vi "Model-free setpoint control0216.vi"() -> ()   [LabVIEW 2018]
doc: "Demonstrates the use of the Network Streams functions to send LED status to the myRIO target."
uses:
  <vilib>/ErrorRing/Error Ring.xnode
  <vilib>/vision/NI_Vision_Development_Module.lvlib
panel:
  in  "base_pr":dbl=-37.75
  in  "base_dr":dbl=-62.3
  in  "K2":dbl=0.109
  in  "K1":dbl=0.138
  in  "Operation":T1(ring)=enum."Erode"
  out "real_relative_point_y":dbl
  out "real_relative_point_x":dbl
  out "real_relative_start_point_y":dbl
  out "real_relative_start_point_x":dbl
  out "Bounding Box.Y Top 2":i32
  out "Bounding Box.X Left 2":i32
  out "Ki part":dbl
  out "Kd part":dbl
  out "Kp part":dbl
  out "Ki part":dbl
  out "Kd part":dbl
  out "Kp part":dbl
  in  "Ki":dbl=0.002
  in  "Kd":dbl=1e-05
  in  "Kp":dbl=0.005
  in  "Ki":dbl=0.002
  in  "Kd":dbl=1e-05
  in  "Kp":dbl=0.005
  out "添加的数组":dbl[](array[numeric])
  in  "desired_relative_point_y":dbl=500.0
  in  "desired_relative_point_x":dbl=400.0
  out "predicted_output_pr":dbl=20.0
  out "predicted_output_dr":dbl=8.0
  out "error_relative_point_y":dbl
  out "error_relative_point_x":dbl
  out "real_relative_end_point_y":dbl
  out "real_relative_end_point_x":dbl
  out "magnet_input_pr":dbl
  out "magnet_input_dr":dbl
  in  "打开仅尖端轨迹":bool
  out "仅尖端轨迹":T2(plugin-control)
  out "Bounding Box.Y Top":i32
  out "Bounding Box.X Left":i32
  out "curve_min_y":dbl
  out "curve_min_x":dbl
  out "curve_max_y":dbl
  out "curve_max_x":dbl
  out "relative_end_point_y":dbl
  out "relative_end_point_x":dbl
  out "delta_y":dbl
  out "delta_x":dbl
  out "pr":dbl
  out "tan(v)":dbl
  out "delta_velocity":dbl format="%#_10g"
  out "delta_time":dbl
  out "now time":timestamp[](array[timestamp])
  out "prev time":timestamp[](array[timestamp])
  out "delta_distance":dbl
  out "prev_end_point_y":dbl
  out "prev_end_point_x":dbl
  out "now_end_point_y":dbl
  out "now_end_point_x":dbl
  out "prev_end_point_y":dbl[](array[numeric])
  out "prev_end_point_x":dbl[](array[numeric])
  out "dr":dbl
  in  "Ar":sgl=11.0
  out "all parameters":dbl[][](array[numeric])
  out "direction angle":sgl[](array[numeric])
  out "dr":sgl
  out "strength":dbl[](array[numeric])
  out "场强":dbl
  out "end_point_y":T3
  out "end_point_x":dbl[](array[numeric])
  out "start_point_y":dbl[](array[numeric])
  out "start_point_x":dbl[](array[numeric])
  out "T":i32[](array[numeric])
  out "c":dbl[](array[numeric])
  out "b":dbl[](array[numeric])
  out "a\na":dbl[](array[numeric])
  out "c":dbl
  out "b":dbl
  out "a":dbl
  out "Angles (deg)":sgl[](array[numeric]) format="%.2f"
  in  "wr":sgl
  in  "打开轨迹":bool
  out "中心轨迹和尖端轨迹":T2(plugin-control)
  out "end_y":dbl
  out "end_x":dbl
  out "start_y":dbl
  out "start_x":dbl
  out "Image Pixels (U8)":u8[][](array[numeric])
  in  "Poly":dbl
  out "中心轨迹":T2(plugin-control)
  in  "保存按钮":bool
  out "Object Center":cluster{"X":sgl, "Y":sgl}
  out "黑白图":T2(plugin-control)
  in  "Number of Erosion":i32=5
  in  "Settings":T4={"Objects"=1, "Threshold"=128, "Reject Border"=FALSE, "Fill Holes"=FALSE, "Min Object Size"=TRUE, "Min Size"=5500, "Max Object Size"=FALSE, "Max Size"=100, "Show Search Area"=TRUE, "Show Center"=TRUE, "Show Bounding Box"=TRUE} {"Objects" items=["Bright Objects", "Dark Objects"]; "Threshold" min=1 max=999999999 step=1; "Max Size" min=1 max=999999999 step=1; "Min Size" min=1 max=999999999 step=1}
  out "Objects":T5(array[cluster]) {"Aspect Ratio" format="%.2f"; "Orientation" format="%.2f"; "Area" format="%.2f"; "Object Center"."Y" format="%.2f"; "Object Center"."X" format="%.2f"}
  in  "Search Rect (entire image)":T6={"Left"=160, "Top"=740, "Right"=1900, "Bottom"=1620, "Rotation"=0.0} {"Rotation" format="%.2f"; "Left" scale=0.0..1024.0; "Right" scale=0.0..1024.0}
  in  "Range":cluster{"Lower value":sgl, "Upper value":sgl}={"Lower value"=170.0, "Upper value"=255.0} {"Upper value" format="%.2f"; "Lower value" format="%.2f"}
  out "原图":T2(plugin-control)
  in  "停止":bool
  out "T":i32
  out "T":i32
  in  "磁场变换":bool=TRUE
  in  "Pause":bool
  out "Array":dbl[](array[numeric])
  in  "Parameter Settings":T7(tab)=enum."Rotating Field" caption="Field Types"
  in  "Ag":dbl
  in  "dg":dbl
  in  "pg":dbl
  in  "fg":dbl
  in  "AoOF":dbl
  in  "fo":sgl
  in  "do":sgl
  in  "oo":sgl
  in  "po":sgl
  in  "cc":sgl
  in  "pc":sgl
  in  "wc":sgl
  in  "dc":sgl
  in  "Ac":dbl
  in  "Dis phase step":dbl
  in  "Dis phase frequency (Hz)":dbl
  in  "Dis tumbling frequency (Hz)":dbl
  in  "Dis strength(mT)":dbl
  in  "Swa strength (mT)":dbl
  in  "Swa frequency (Hz)":dbl
  in  "Swa pitch angle (deg)":dbl
  in  "Swa direction angle (deg)":dbl
  in  "Swa ratio":dbl=1.0
  in  "Pitch Angle (rotating around Constant, deg)":dbl
  in  "Ratio (A/C)":sgl
  in  "Direction Angle (deg)":sgl
  in  "Pitch Angle (rotating around Origin, deg)":sgl
  in  "Frequency (Hz)":sgl
  in  "Strength (mT)":dbl
  in  "Ar 2":dbl caption="Ar"
  in  "ratio":sgl
  in  "pr  2":sgl
  in  "dr  2":sgl
  in  "wr  2":sgl
  in  "p_x":sgl
  out "Numeric 5":i32
  in  "Stop":bool
  out "error out":errorcluster
  in  "Target IP Address":string="172.22.11.2"
  # "Overview: Magnetic field calculation, and send parameters to myRIO\nInstructions:\n1. Verify the value of Target IP Address. Set Visa resource name.\n2. Ensure RT Main.vi is already running. \n3. Run this VI. Set parameters of magnetic field."
  # "Strength (mT)"
  # "Frequency (Hz)"
  # "Pitch Angle (deg)"
  # "Direction Angle (deg)"
  # "Strength (mT)"
  # "Pitch Angle (deg)"
  # "Direction Angle (deg)"
  # "Frequency (Hz)"
  # "Strength (mT)"
  # "Oscilation Frequency (Hz)"
  # "Oscilation Angle (deg)"
  # "Pitch Angle (deg)"
  # "Direction Angle (deg)"
  # "Strength (mT)"
  # "Frequency (Hz)"
  # "Pitch Angle (deg)"
  # "Direction Angle (deg)"
  # "Conical Angle (deg)"
  # "Strength (mT)"
  # "Tumbling Frequency (Hz)"
  # "Phase Frequency (Hz)"
  # "Phase Step"
  # "Strength (mT)"
  # "Frequency (Hz)"
  # "Pitch Angle (deg)"
  # "Direction Angle (deg)"
  # "Ratio"
  # "Strength (mT)"
  # "Frequency (Hz)"
  # "Ratio (A/C)"
  # "Direction Angle (deg)"
  # "Pitch Angle (rotating around Origin, deg)"
  # "Pitch Angle (rotating around Constant, deg)"
  # "Strength (mT)"
  # "Frequency (Hz)"
  # "Pitch Angle Y (deg)"
  # "Pitch Angle X (deg)"
  # "Direction Angle (deg)"
  # "ratio (l/s)"
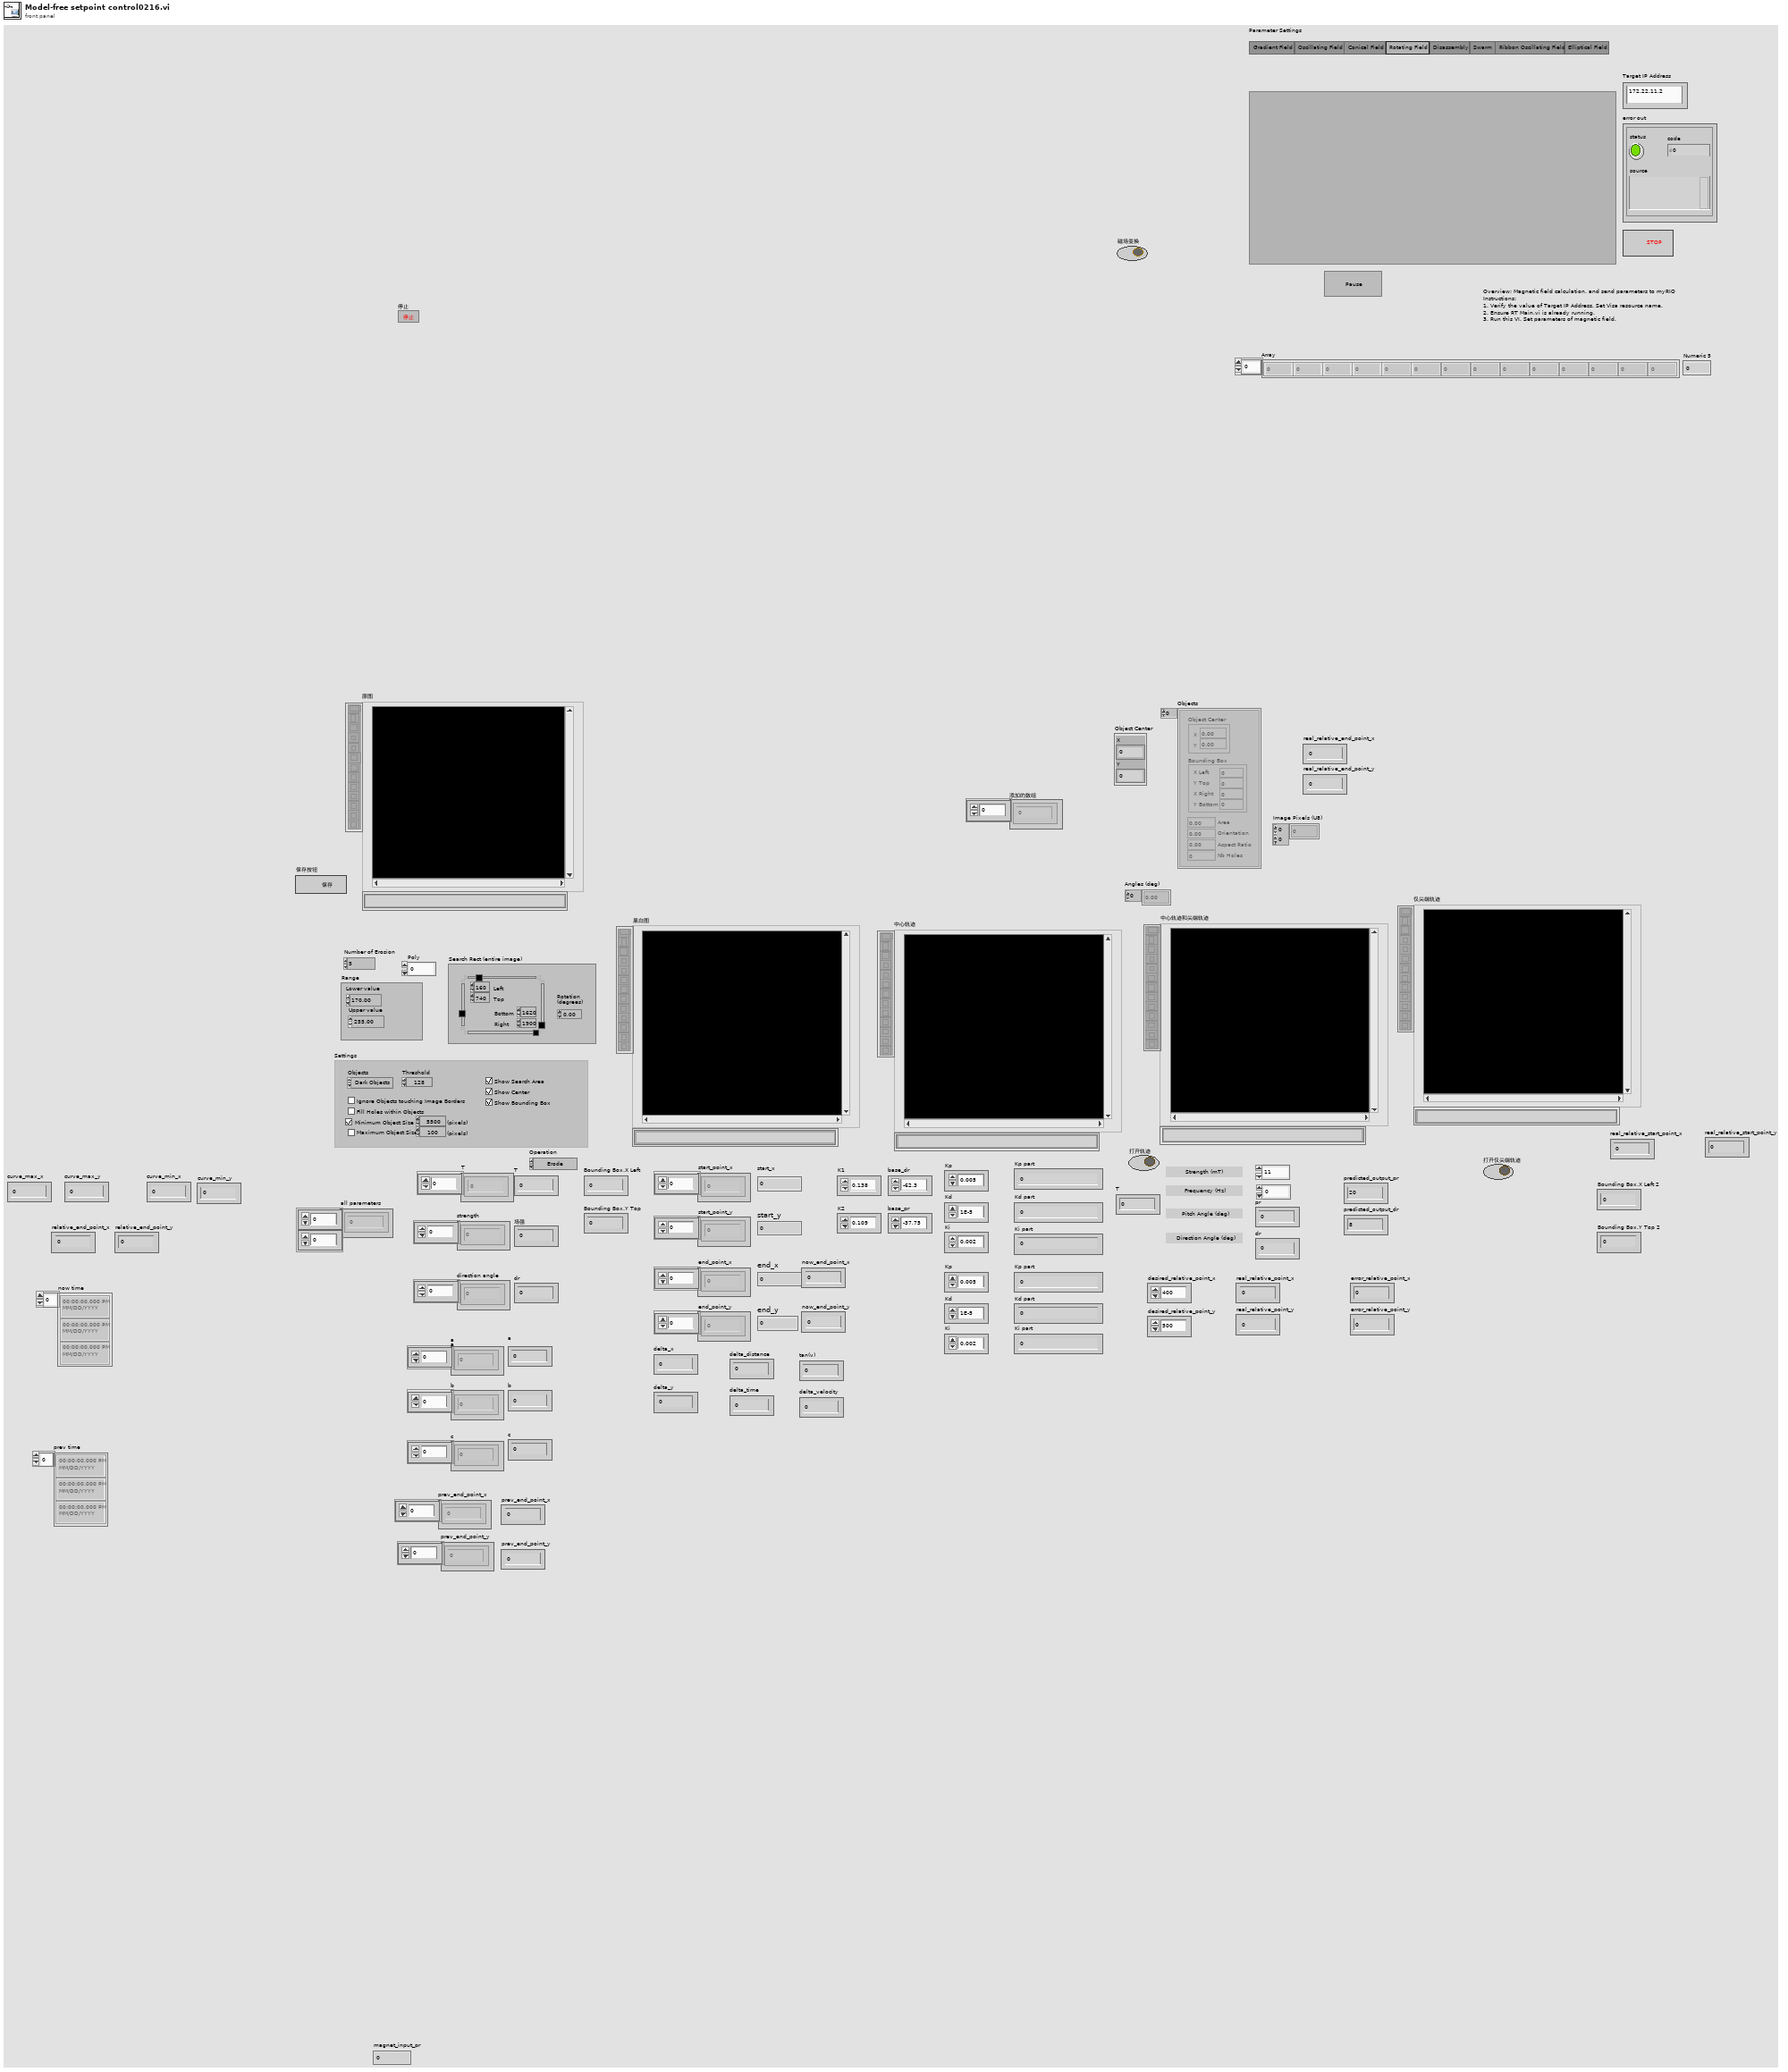
[diagram p1: front panel]
types:
  T1 = enum32{"AutoM", "Close", "Dilate", "Erode", "Gradient", "Gradient in", "Gradient out", "HitMiss", "Open", "PClose", "POpen", "Thick", "Thin"}
  T2 = typedef "IMAQ Image.ctl" = refnum<image>
  T3 = typedef "控件 3.ctl" = dbl[]
  T4 = cluster{"Objects":u16, "Threshold":i32, "Reject Border":bool, "Fill Holes":bool, "Min Object Size":bool, "Min Size":i32, "Max Object Size":bool, "Max Size":i32, "Show Search Area":bool, "Show Center":bool, "Show Bounding Box":bool}
  T5 = cluster{"Object Center":cluster{"X":sgl, "Y":sgl}, "Bounding Box":cluster{"X Left":i32, "Y Top":i32, "X Right":i32, "Y Bottom":i32}, "Area":sgl, "Orientation":sgl, "Aspect Ratio":sgl, "Nb Holes":i32}[]
  T6 = typedef "IMAQ Rectangle" = cluster{"Left":i32, "Top":i32, "Right":i32, "Bottom":i32, "Rotation":dbl}
  T7 = enum32{"Gradient Field ", "Oscillating Field", "Conical Field", "Rotating Field", "Disassembly", "Swarm", "Ribbon Oscillating Field", "Elliptical Field"}
  T8 = typedef "Image Type" = u32
  T9 = cluster{"Object Center":cluster{"X":sgl, "Y":sgl}, "Bounding Box":cluster{"X Left":i32, "Y Top":i32, "X Right":i32, "Y Bottom":i32}, "Area":sgl, "Orientation":sgl, "Aspect Ratio":sgl, "Nb Holes":i32}
  T10 = cluster{"X Left":i32, "Y Top":i32, "X Right":i32, "Y Bottom":i32, "Rotation":dbl}
  T11 = typedef "ROI Descriptor" = cluster{"Global Rectangle":i32[], "Contours":cluster{"ID":enum32{"External", "Internal"}, "Type":u32, "Coordinates":i32[]}[]}
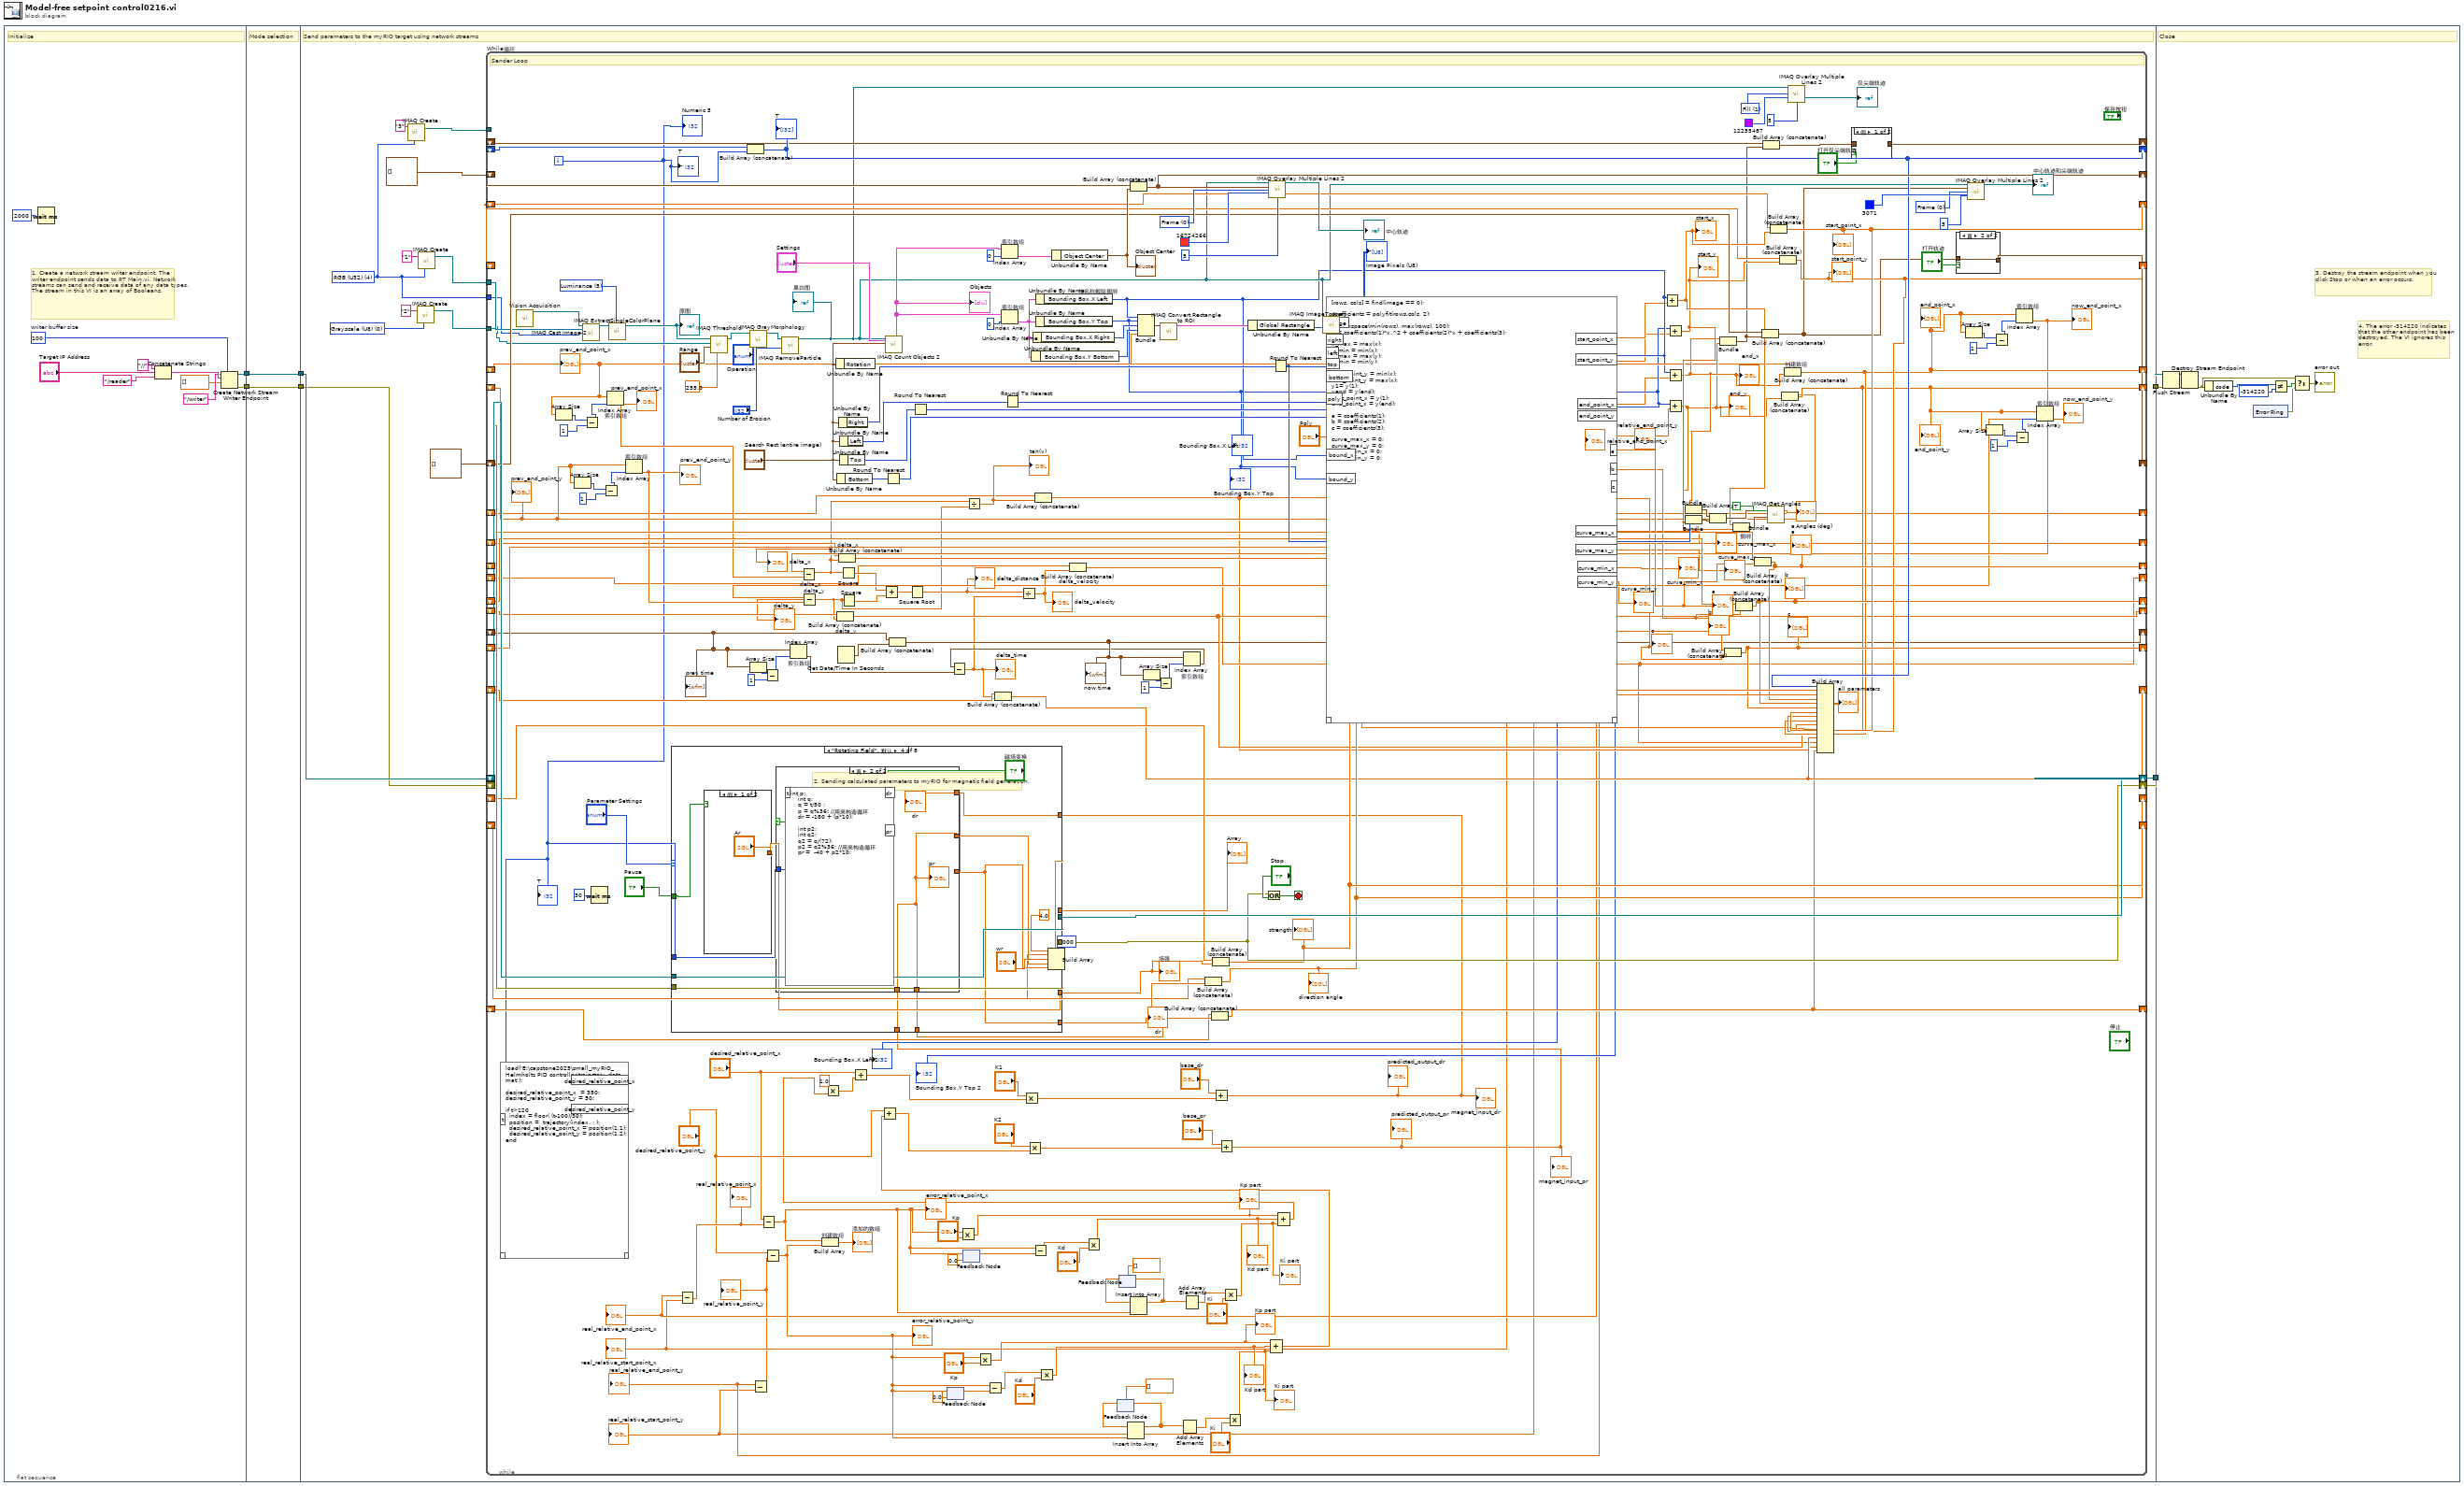
[diagram p0: block diagram]
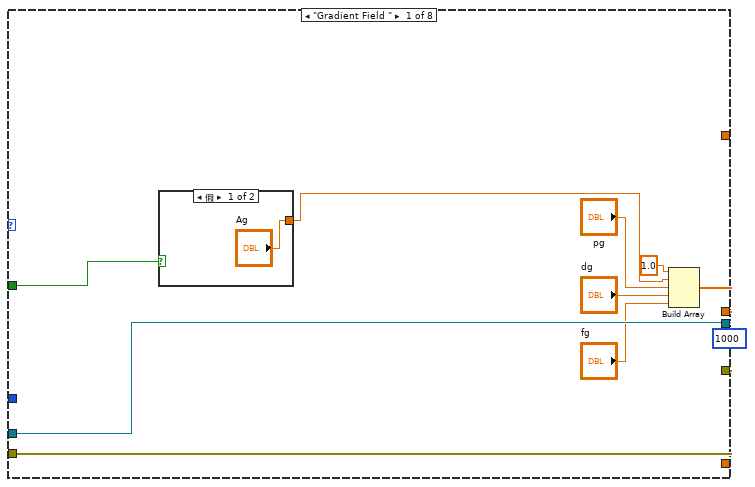
[diagram p4: hidden frame]
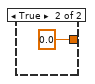
[diagram p5: hidden frame]
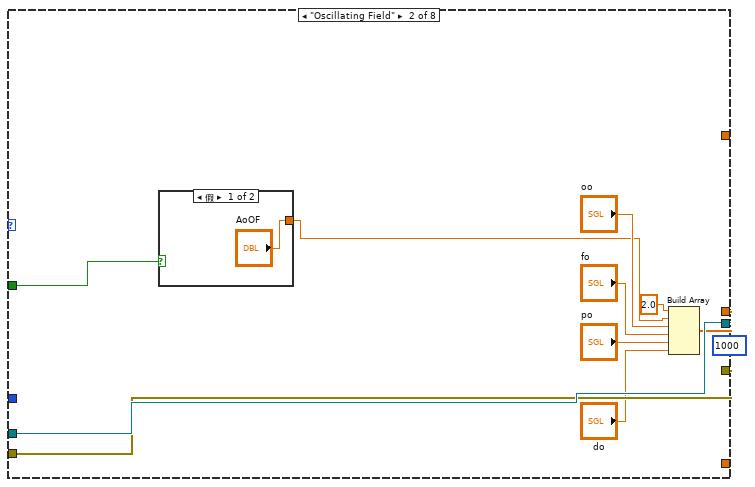
[diagram p6: hidden frame]
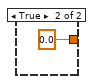
[diagram p7: hidden frame]
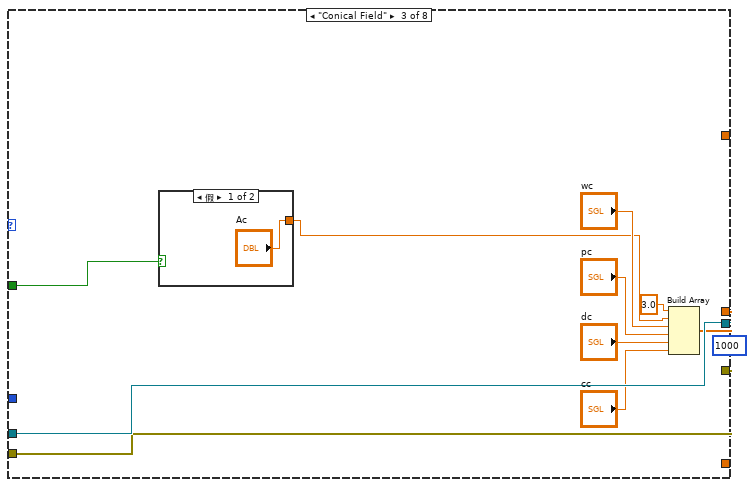
[diagram p8: hidden frame]
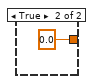
[diagram p9: hidden frame]
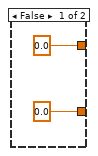
[diagram p10: hidden frame]
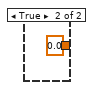
[diagram p11: hidden frame]
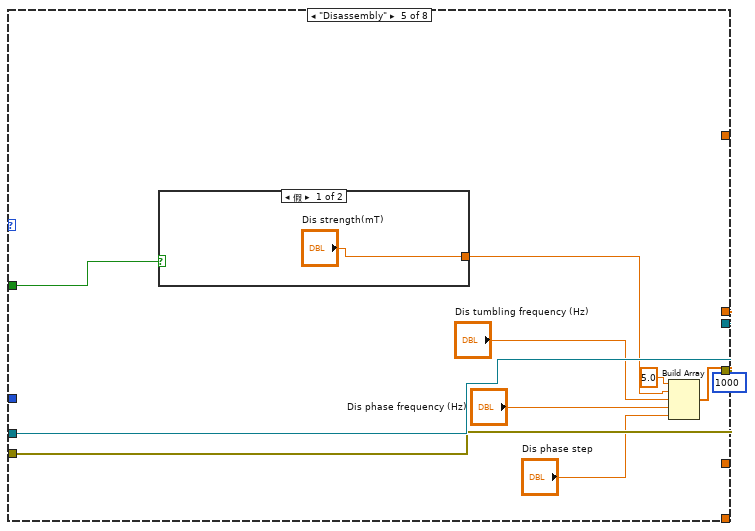
[diagram p12: hidden frame]
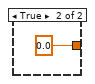
[diagram p13: hidden frame]
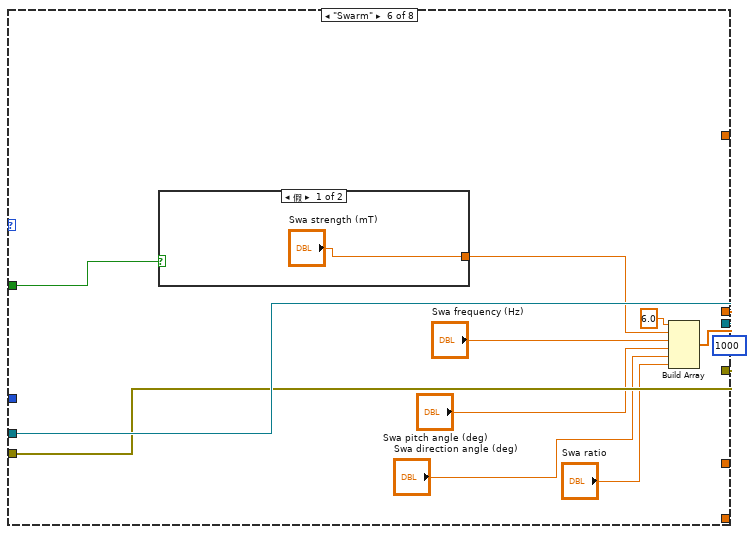
[diagram p14: hidden frame]
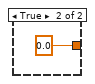
[diagram p15: hidden frame]
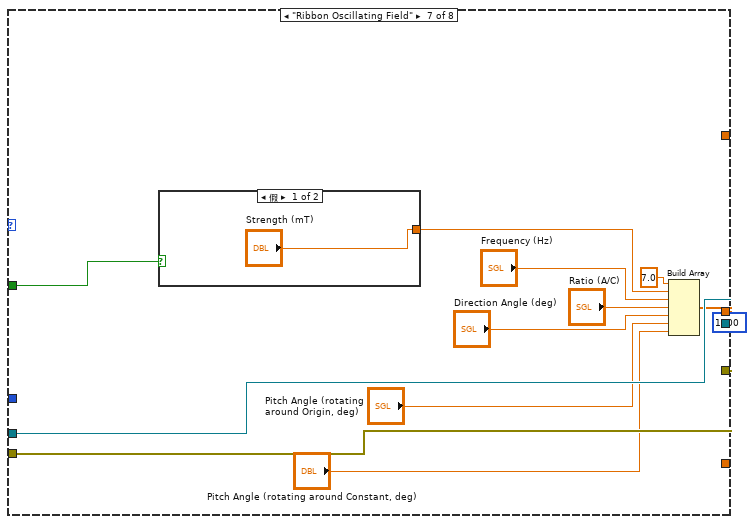
[diagram p16: hidden frame]
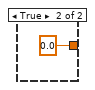
[diagram p17: hidden frame]
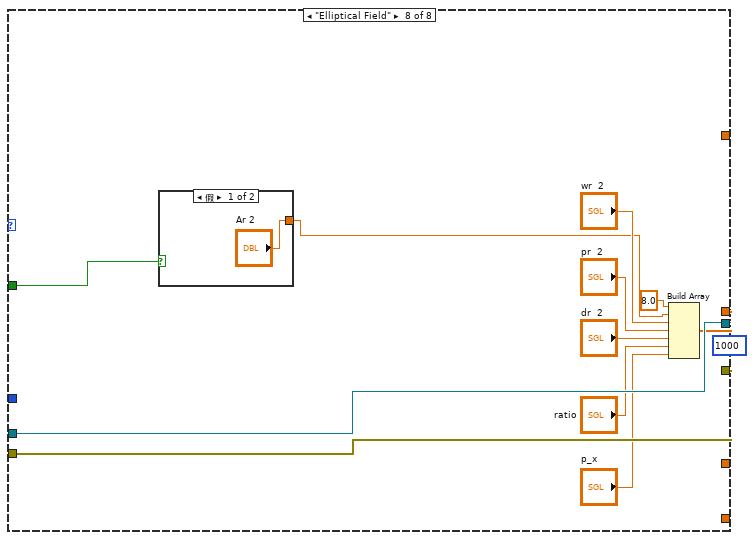
[diagram p18: hidden frame]
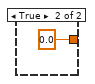
[diagram p19: hidden frame]
diagram:
  n1 = flat-sequence {
    tunnel: [w11] -> w2
    tunnel: [w10] -> w1
    tunnel: [w18] -> w4
    tunnel: [w17] -> w3
    tunnel: w1 -> [w17]
    tunnel: w2 -> [w18]
    tunnel: [w30] -> w6
    tunnel: w4 -> [w32]
    tunnel: [w29] -> w5
    tunnel: w3 -> [w31]
    tunnel: w6 -> [w387]
    tunnel: w5 -> [w384]
    frame #0 {
      w9 = 100  # writer buffer size
      # "1. Create a network stream writer endpoint. The writer endpoint sends data to RT Main.vi. Network streams can send and receive data of any data types. The stream in this VI is an array of Booleans."
      # "Initialize"
      n2 = Wait (ms)(milliseconds to wait=2000) -> ()  [unwired: 1 out]
      n3 = Concatenate Strings("//", "Target IP Address", "/reader") -> (w16:string)
      n4 = Create Network Stream Writer Endpoint(7:w9, 9:dbl[] [], 10:w16, 11:"/writer" ("reader name")) -> (0:w10:errorcluster, 3:w11:refnum<k21>)  [unwired: 3 in]
    }
    frame #1 {
      # "Mode selection"
    }
    frame #2 {
      w26 = T8 0 items=["Grayscale (U8)", "Grayscale (I16)", "Grayscale (SGL)", "Complex (CSG)", "RGB (U32)", "HSL (U32)", "RGB (U64)", "Grayscale (U16)"] ("Image Type")
      w19 = T8 4 items=["Grayscale (U8)", "Grayscale (I16)", "Grayscale (SGL)", "Complex (CSG)", "RGB (U32)", "HSL (U32)", "RGB (U64)", "Grayscale (U16)"] ("Image Type")
      # "Send parameters to the myRIO target using network streams"
      n5 = call "IMAQ Create"("Image Name"="3", "Image Type"=w19) -> ("New Image"=w22:T2)  [unwired: 3 in, 1 out]
      n6 = call "IMAQ Create"("Image Name"="2", "Image Type"=w26) -> ("New Image"=w24:T2)  [unwired: 3 in, 1 out]
      n7 = call "IMAQ Create"("Image Name"="1", "Image Type"=w19) -> ("New Image"=w25:T2)  [unwired: 3 in, 1 out]
      n8 = while "While循环" {
        shift-right: [w242] -> w29
        shift-left: w31 -> [w244]
        shift-right: [w243] -> w30
        shift-left: w32 -> [w245]
        tunnel: w25 -> [w196]
        tunnel: w24 -> [w195]
        tunnel: w22 -> [_]
        shift-right: [w192] -> _
        shift-left: cluster{"X":dbl, "Y":dbl}[] [] -> [w197]
        shift-right: [w198] -> _
        shift-left: cluster{"X":dbl, "Y":dbl}[] [] -> [w199]
        tunnel: w19 -> [w194]
        shift-right: [w164] -> _
        shift-left: _ -> [w184]
        shift-right: [w159] -> _
        shift-left: _ -> [w182]
        shift-right: [w163] -> _
        shift-left: _ -> [w179]
        shift-right: [w167] -> _
        shift-left: _ -> [w178]
        shift-right: [w162] -> _
        shift-left: _ -> [w176]
        shift-right: [w161] -> _
        shift-left: _ -> [w174]
        shift-right: [w155] -> _
        shift-left: _ -> [w147]
        shift-right: [w151] -> _
        shift-left: _ -> [w143]
        shift-right: [w166] -> _
        shift-left: _ -> [w170]
        shift-right: [w165] -> _
        shift-left: _ -> [w168]
        shift-right: [w132] -> _
        shift-left: _ -> [w134]
        shift-right: [w131] -> _
        shift-left: _ -> [w133]
        shift-right: [w121] -> _
        shift-left: _ -> [w126]
        shift-right: [w118] -> _
        shift-left: _ -> [w119]
        shift-right: [w114] -> _
        shift-left: _ -> [w115]
        shift-right: [w109] -> _
        shift-left: _ -> [w110]
        shift-right: [w101] -> _
        shift-left: _ -> [w102]
        shift-right: [w95] -> _
        shift-left: _ -> [w96]
        i -> [w89]
        stop <- w238 stop-if-true
        w97 = u32 1 items=["Frame", "Fill"] ("Drawing Mode (Frame)")
        w104 = u32 0 items=["Frame", "Fill"] ("Drawing Mode (Frame)")
        w225 = u32 0 items=["Frame", "Fill"] ("Drawing Mode (Frame)")
        w235 = 5 items=["Red", "Green", "Blue", "Hue", "Saturation", "Luminance", "Value", "Intensity"] ("Color Plane")
        # "2. Sending calculated parameters to myRIO for magnetic field generation."
        # "Sender Loop"
        n9 = script code="load('E:\\capstone2025\\small_myRIO_Helmholtz PID controller\\trajectory_data.mat');\n\ndesired_relative_point_x  = 350;\ndesired_relative_point_y = 50;\n\nif t>120\n  index = floor( (t-100)/30);\n  position =  trajectory(index, : );\n  desired_relative_point_x = position(1,1);\n  desired_relative_point_y = position(1,2);\nend"("t"=w89) -> ()  [unwired: 1 in, 3 out]
        n10 = call "Vision Acquisition"() -> ("Image Out"=w223:T2)  [unwired: 23 in, 4 out]
        n11 = Array Size(array=w147) -> (size(s)=w149:i32)
        n12 = Array Size(array=w143) -> (size(s)=w145:i32)
        n13 = call "IMAQ Cast Image 2"("Image Src"=w223, "Image Dst"=w196, "Image Type"=w194) -> ("Image Dst Out"=w236:T2)  [unwired: 11 in, 1 out]
        n14 = Subtract(x=w149, y=1) -> (x-y=w148:i32)
        n15 = Wait (ms)(milliseconds to wait=u32 30 ("等待时间（毫秒）")) -> ()  [unwired: 1 out]
        n16 = Subtract(x=w145, y=1) -> (x-y=w144:i32)
        n17 = Index Array "索引数组"(array=w147, index=w148) -> (element=w141:dbl)
        "prev_end_point_x" <- w141
        n18 = call "IMAQ ExtractSingleColorPlane"("Color Plane"=w235, "Image Src"=w236) -> ("Image Dst Out"=w234:T2)  [unwired: 8 in, 1 out]
        "原图" <- w234
        n19 = Index Array "索引数组"(array=w143, index=w144) -> (element=w140:dbl)
        "prev_end_point_y" <- w140
        n20 = call "IMAQ Threshold"("Replace Value"=sgl 255.0, "Range"="Range", "Image Dst"=w195, "Image Src"=w234) -> ("Image Dst Out"=w50:T2)  [unwired: 6 in, 1 out]
        n21 = Build Array (concatenate)(w178, w89) -> (w167:i32[])
        "T" <- w167
        n22 = call "IMAQ GrayMorphology"("Operation"="Operation", "Image Src"=w50) -> ("Image Dst Out"=w49:T2)  [unwired: 8 in, 1 out]
        n23 = Array Size(array=w126) -> (size(s)=w129:i32)
        n24 = Subtract(x=w129, y=1) -> (x-y=w128:i32)
        n25 = call "IMAQ RemoveParticle"("Number of Erosion"="Number of Erosion", "Image Src"=w49) -> ("Image Dst Out"=w93:T2)  [unwired: 8 in, 1 out]
        "黑白图" <- w93
        n26 = Index Array "索引数组"(array=w126, index=w128) -> (element=w125:timestamp)
        n27 = Unbundle By Name("Search Rect (entire image)") -> ("Rotation"=w220:dbl)
        n28 = Unbundle By Name("Search Rect (entire image)") -> ("Bottom"=w204:i32)
        n29 = Get Date/Time In Seconds() -> (seconds since 1Jan1904=w130:timestamp)
        n30 = Unbundle By Name("Search Rect (entire image)") -> ("Right"=w208:i32)
        n31 = Unbundle By Name("Search Rect (entire image)") -> ("Left"=w207:i32)
        n32 = Unbundle By Name("Search Rect (entire image)") -> ("Top"=w206:i32)
        n33 = Round To Nearest(number=w204) -> (nearest integer value=w203:i32)
        n34 = call "IMAQ Count Objects 2"("Settings"="Settings", "Search Rect (entire image)"="Search Rect (entire image)", "Image"=w93) -> ("Objects"=w222:T5)  [unwired: 4 in, 4 out]
        "Objects" <- w222
        n35 = Build Array (concatenate)(w126, w130) -> (w121:timestamp[])
        "now time" <- w121
        n36 = Round To Nearest(number=w206) -> (nearest integer value=w205:i32)
        n37 = feedback #1(0.0) -> (w71:dbl)
        n38 = feedback #2(0.0) -> (w85:dbl)
        n39 = Index Array "索引数组"(array=w222, index=0 ("索引")) -> (element=w228:T9)
        n40 = Index Array "索引数组"(array=w222, index=0 ("索引")) -> (element=w218:T9)
        n41 = Round To Nearest(number=w207) -> (nearest integer value=w201:i32)
        n42 = Unbundle By Name(w218) -> ("Bounding Box.Y Bottom"=w212:i32)
        n43 = Unbundle By Name(w218) -> ("Bounding Box.X Right"=w213:i32)
        n44 = Unbundle By Name "按名称解除捆绑"(w218) -> ("Bounding Box.X Left"=w58:i32)
        "Bounding Box.X Left" <- w58
        "Bounding Box.X Left 2" <- w58
        n45 = Unbundle By Name(w218) -> ("Bounding Box.Y Top"=w57:i32)
        "Bounding Box.Y Top" <- w57
        "Bounding Box.Y Top 2" <- w57
        n46 = Unbundle By Name(w228) -> ("Object Center"=w227:cluster{"X":sgl, "Y":sgl})
        "Object Center" <- w227
        n47 = feedback #3(dbl[] []) -> (w66:dbl[])
        n48 = feedback #4(dbl[] []) -> (w80:dbl[])
        n49 = Build Array (concatenate)(w199, w227) -> (w198:cluster{"X":dbl, "Y":dbl}[])
        n50 = Bundle("X Left"=w58, "Y Top"=w57, "X Right"=w213, "Y Bottom"=w212, "Rotation"=w220) -> (w219:T10)  [unwired: 1 in]
        n51 = Array Size(array=w121) -> (size(s)=w124:i32)
        n52 = Subtract(x=w124, y=1) -> (x-y=w123:i32)
        n53 = call "IMAQ Convert Rectangle to ROI"("Rectangle"=w219) -> ("ROI Descriptor"=w217:T11)  [unwired: 8 in, 1 out]
        n54 = Index Array "索引数组"(array=w121, index=w123) -> (element=w120:timestamp)
        n55 = Subtract(x=w120, y=w125) -> (x-y=w117:dbl)
        "delta_time" <- w117
        n56 = Build Array (concatenate)(w119, w117) -> (w118:dbl[])
        n57 = Unbundle By Name(w217) -> ("Global Rectangle"=w202:i32[])
        n58 = call "IMAQ Overlay Multiple Lines 2"("Image"=w93, "Line End Points"=w198, "Drawing Mode (Frame)"=w225, "Color"=u32 16724266, "Width"=u32 5) -> ("Image Out"=→"中心轨迹":T2)  [unwired: 9 in, 1 out]
        n59 = Round To Nearest(number=w208) -> (nearest integer value=w185:i32)
        n60 = call "IMAQ ImageToArray"("Optional Rectangle"=w202, "Image"=w93) -> ("Image Pixels (U8)"=w214:u8[][])  [unwired: 2 in, 4 out]
        "Image Pixels (U8)" <- w214
        n61 = script code="[rows, cols] = find(image == 0); \n\ncoefficients = polyfit(rows,cols, 2);\n\nx = linspace(min(rows), max(rows), 100); \ny = coefficients(1)*x.^2 + coefficients(2)*x + coefficients(3);\n\nx_max = max(x);\nx_min = min(x);\ny_max = max(y);\ny_min = min(y);\n\nstart_point_y = min(x);\nend_point_y = max(x);\ny1= y(1);\nyend = y(end);\nstart_point_x = y(1);\nend_point_x = y(end);\n\na = coefficients(1);\nb = coefficients(2);\nc = coefficients(3);\n\ncurve_max_x = 0;\ncurve_max_y = 0;\ncurve_min_x = 0;\ncurve_min_y = 0;"("image"=w214, "poly"="Poly", "right"=w185, "left"=w201, "top"=w205, "bottom"=w203, "bound_x"=w58, "bound_y"=w57) -> ("start_point_x"=w55:dbl, "start_point_y"=w52:dbl, "end_point_x"=w56:dbl, "end_point_y"=w53:dbl, "a"=w183:dbl, "b"=w181:dbl, "c"=w180:dbl, "curve_max_x"=→"curve_max_x":dbl, "curve_max_y"=→"curve_max_y":dbl, "curve_min_x"=→"curve_min_x":dbl, "curve_min_y"=→"curve_min_y":dbl)  [unwired: 1 in, 1 out]
        "a" <- w183
        "b" <- w181
        "c" <- w180
        "relative_end_point_x" <- w56
        "relative_end_point_y" <- w53
        "real_relative_end_point_x" <- w56
        "real_relative_end_point_y" <- w53
        "real_relative_start_point_x" <- w55
        "real_relative_start_point_y" <- w52
        n62 = Subtract(x=w56, y=w55) -> (x-y=w54:dbl)
        "real_relative_point_x" <- w54
        n63 = Subtract(x=w53, y=w52) -> (x-y=w51:dbl)
        "real_relative_point_y" <- w51
        n64 = Subtract(x="desired_relative_point_x", y=w54) -> (x-y=w79:dbl)
        "error_relative_point_x" <- w79
        n65 = Subtract(x="desired_relative_point_y", y=w51) -> (x-y=w64:dbl)
        "error_relative_point_y" <- w64
        n66 = Build Array "创建数组"(w79, w64) -> (→"添加的数组":dbl[])
        n67 = feedback-in #1(w64) -> ()
        n68 = Multiply(x=w79, y="Kp") -> (x*y=w86:dbl)
        "Kp part" <- w86
        n69 = feedback-in #2(w79) -> ()
        n70 = Multiply(x=w64, y="Kp") -> (x*y=w72:dbl)
        "Kp part" <- w72
        n71 = Subtract(x=w64, y=w71) -> (x-y=w69:dbl)
        n72 = Subtract(x=w79, y=w85) -> (x-y=w83:dbl)
        n73 = Multiply(x=w69, y="Kd") -> (x*y=w67:dbl)
        "Kd part" <- w67
        n74 = Multiply(x=w83, y="Kd") -> (x*y=w81:dbl)
        "Kd part" <- w81
        n75 = Insert Into Array(array=w66, new element=w64) -> (w65:dbl[])  [unwired: 1 in]
        n76 = feedback-in #3(w65) -> ()
        n77 = Insert Into Array(array=w80, new element=w79) -> (w78:dbl[])  [unwired: 1 in]
        n78 = feedback-in #4(w78) -> ()
        n79 = Add Array Elements(numeric array=w65) -> (sum=w62:dbl)
        n80 = Add Array Elements(numeric array=w78) -> (sum=w76:dbl)
        n81 = Multiply(x=w76, y="Ki") -> (x*y=w74:dbl)
        "Ki part" <- w74
        n82 = Multiply(x=w62, y="Ki") -> (x*y=w60:dbl)
        "Ki part" <- w60
        n83 = Compound Arithmetic op=ADD(w72, w67, w60) -> (w59:dbl)
        n84 = Add(x="desired_relative_point_y", y=w59) -> (x+y=w45:dbl)
        n85 = Multiply(x="K2", y=w45) -> (x*y=w40:dbl)
        n86 = Add(x="base_pr", y=w40) -> (x+y=w38:dbl)
        "magnet_input_pr" <- w38
        "predicted_output_pr" <- w38
        n87 = Compound Arithmetic op=ADD(w86, w81, w74) -> (w35:dbl)
        n88 = Multiply(x=1.0, y=w35) -> (x*y=w33:dbl)
        n89 = Add(x="desired_relative_point_x", y=w33) -> (x+y=w47:dbl)
        n90 = Multiply(x="K1", y=w47) -> (x*y=w43:dbl)
        n91 = Add(x="base_dr", y=w43) -> (x+y=w42:dbl)
        "magnet_input_dr" <- w42
        "predicted_output_dr" <- w42
        n92 = case shown="\"Rotating Field\", 默认" "Parameter Settings" {
          tunnel: w245 -> [w259 w274 w289 w308 w327 w341 w359 w374]
          tunnel: w244 -> [w256 w273 w288 w307 w325 w340 w357 w373]
          tunnel: [w258 w272 w286 w306 w326 w339 w358 w372] -> w243
          tunnel: [w257 w271 w287 w305 w324 w338 w356 w371] -> w242
          tunnel: [w252 w265 w280 w301 w318 w333 w354 w366] -> w241
          tunnel: "Pause" -> [w250 w263 w278 w300 w317 w332 w349 w364]
          tunnel: [_ _ _ w297 _ _ _ _] -> w171
          tunnel: [_ _ _ w298 _ _ _ _] -> w169
          tunnel: w89 -> [_ _ _ w296 _ _ _ _]
          tunnel: [_ _ _ w295 _ _ _ _] -> w103
          tunnel: w42 -> [_ _ _ w294 _ _ _ _]
          tunnel: w38 -> [_ _ _ w293 _ _ _ _]
          frame "Gradient Field " {
            n93 = case shown="假" w250 {
              tunnel: ["Ag" 0.0] -> w251
              frame False {
              }
              frame True {
              }
            }
            n94 = Build Array(1.0, w251, "pg", "dg", "fg") -> (w252:dbl[])
            n95 = shared-variable-write(w259, w256, w252, 1000 ("timeout ms (-1)")) -> (w258:refnum<k21>, w257:errorcluster)  [unwired: 1 out]
          }
          frame "Oscillating Field" {
            n96 = case shown="假" w263 {
              tunnel: ["AoOF" 0.0] -> w264
              frame False {
              }
              frame True {
              }
            }
            n97 = Build Array(2.0, w264, "oo", "fo", "po", "do") -> (w265:dbl[])
            n98 = shared-variable-write(w274, w273, w265, 1000 ("timeout ms (-1)")) -> (w272:refnum<k21>, w271:errorcluster)  [unwired: 1 out]
          }
          frame "Conical Field" {
            # "FG"
            n99 = case shown="假" w278 {
              tunnel: ["Ac" 0.0] -> w279
              frame False {
              }
              frame True {
              }
            }
            n100 = Build Array(3.0, w279, "wc", "pc", "dc", "cc") -> (w280:dbl[])
            n101 = shared-variable-write(w289, w288, w280, 1000 ("timeout ms (-1)")) -> (w286:refnum<k21>, w287:errorcluster)  [unwired: 1 out]
          }
          frame "Rotating Field", Default {
            n102 = case shown="假" w300 {
              tunnel: ["Ar" 0.0] -> w297
              frame False {
              }
              frame True {
              }
            }
            n103 = case shown="真" "磁场变换" {
              tunnel: [sgl 0.0 ("pr") w312] -> w303
              tunnel: [sgl 0.0 ("dr") w313] -> w298
              tunnel: w296 -> [_ w314]
              tunnel: [_ w312] -> w295
              tunnel: w294 -> [_ w313]
              tunnel: w293 -> [_ w312]
              frame False {
              }
              frame True {
                n104 = formula code="int p;\n    int q;\n    q = t/50 ;  \n    p = q%36; //用来构造循环\n    dr = -180 + (p*10);\n\n    int p2;\n    int q2;\n    q2 = q/(72);\n    p2 = q2%36; //用来构造循环\n    pr =  -40 + p2*10;"("t"=w314) -> ()  [unwired: 2 out]
                "dr" <- w313
                "pr" <- w312
              }
            }
            n105 = Build Array(4.0, w297, "wr", w303, w298) -> (w301:dbl[])
            n106 = shared-variable-write "向流中写入单个元素"(w308, w307, w301, 1000 ("timeout ms (-1)")) -> (w306:refnum<k21>, w305:errorcluster)  [unwired: 1 out]
          }
          frame "Disassembly" {
            n107 = case shown="假" w317 {
              tunnel: ["Dis strength(mT)" 0.0] -> w322
              frame False {
              }
              frame True {
              }
            }
            n108 = Build Array(5.0, w322, "Dis tumbling frequency (Hz)", "Dis phase frequency (Hz)", "Dis phase step") -> (w318:dbl[])
            n109 = shared-variable-write(w327, w325, w318, 1000 ("timeout ms (-1)")) -> (w326:refnum<k21>, w324:errorcluster)  [unwired: 1 out]
          }
          frame "Swarm" {
            n110 = case shown="假" w332 {
              tunnel: ["Swa strength (mT)" 0.0] -> w331
              frame False {
              }
              frame True {
              }
            }
            n111 = Build Array(6.0, w331, "Swa frequency (Hz)", "Swa pitch angle (deg)", "Swa direction angle (deg)", "Swa ratio") -> (w333:dbl[])
            n112 = shared-variable-write(w341, w340, w333, 1000 ("timeout ms (-1)")) -> (w339:refnum<k21>, w338:errorcluster)  [unwired: 1 out]
          }
          frame "Ribbon Oscillating Field" {
            n113 = case shown="假" w349 {
              tunnel: ["Strength (mT)" 0.0] -> w348
              frame False {
              }
              frame True {
              }
            }
            n114 = Build Array(7.0, w348, "Frequency (Hz)", "Ratio (A/C)", "Direction Angle (deg)", "Pitch Angle (rotating around Origin, deg)", "Pitch Angle (rotating around Constant, deg)") -> (w354:dbl[])
            n115 = shared-variable-write(w359, w357, w354, 1000 ("timeout ms (-1)")) -> (w358:refnum<k21>, w356:errorcluster)  [unwired: 1 out]
          }
          frame "Elliptical Field" {
            n116 = case shown="假" w364 {
              tunnel: ["Ar 2" 0.0] -> w365
              frame False {
              }
              frame True {
              }
            }
            n117 = Build Array(8.0, w365, "wr  2", "pr  2", "dr  2", "ratio", "p_x") -> (w366:dbl[])
            n118 = shared-variable-write(w374, w373, w366, 1000 ("timeout ms (-1)")) -> (w372:refnum<k21>, w371:errorcluster)  [unwired: 1 out]
          }
        }
        "Array" <- w241
        "场强" <- w171
        "dr" <- w169
        n119 = Build Array (concatenate)(w168, w169) -> (w165:dbl[])
        "direction angle" <- w165
        n120 = Build Array (concatenate)(w102, w103) -> (w101:dbl[])
        n121 = Build Array (concatenate)(w170, w171) -> (w166:dbl[])
        "strength" <- w166
        n122 = Or(x=w242, y="Stop") -> (x .or. y?=w238:bool)
        n123 = Add(x=w58, y=w55) -> (x+y=w177:dbl)
        "start_x" <- w177
        n124 = Add(x=w57, y=w52) -> (x+y=w175:dbl)
        "start_y" <- w175
        n125 = Add(x=w58, y=w56) -> (x+y=w173:dbl)
        "end_x" <- w173
        n126 = Add(x=w57, y=w53) -> (x+y=w172:dbl)
        "end_y" <- w172
        n127 = Bundle(w173, w172) -> (w189:cluster{dbl, dbl})  [unwired: 1 in]
        n128 = Bundle(w185, w175) -> (w188:cluster{i32, dbl})  [unwired: 1 in]
        n129 = Build Array(w189, w188) -> (w187:cluster{dbl, dbl}[])
        n130 = Bundle(w173, w172) -> (w91:cluster{dbl, dbl})  [unwired: 1 in]
        n131 = Build Array (concatenate)(w179, w180) -> (w163:dbl[])
        "c" <- w163
        n132 = Bundle "捆绑"(w177, w175) -> (w190:cluster{dbl, dbl})  [unwired: 1 in]
        n133 = Build Array (concatenate)(w182, w181) -> (w159:dbl[])
        "b" <- w159
        n134 = Build Array (concatenate)(w184, w183) -> (w164:dbl[])
        "a\na" <- w164
        n135 = Build Array (concatenate)(w197, w91) -> (w92:cluster{"X":dbl, "Y":dbl}[])
        n136 = Build Array (concatenate)(w96, w91) -> (w90:cluster{dbl, dbl}[])
        n137 = call "IMAQ Get Angles"("Vertex"=w190, "Points"=w187, "Use Vertex (No)"=TRUE) -> ("Angles (deg)"=→"Angles (deg)":sgl[])  [unwired: 2 in, 2 out]
        n138 = Build Array (concatenate)(w176, w177) -> (w162:dbl[])
        "start_point_x" <- w162
        n139 = Build Array (concatenate)(w174, w175) -> (w161:dbl[])
        "start_point_y" <- w161
        n140 = Build Array (concatenate)(w143, w172) -> (w151:dbl[])
        "end_point_y" <- w151
        n141 = Build Array (concatenate) "创建数组"(w147, w173) -> (w155:dbl[])
        "end_point_x" <- w155
        n142 = call "IMAQ Overlay Multiple Lines 2"("Image"=w93, "Drawing Mode (Frame)"=w97, "Color"=u32 12255487, "Width"=u32 5) -> ("Image Out"=→"仅尖端轨迹":T2)  [unwired: 10 in, 1 out]
        n143 = case shown="假" "打开仅尖端轨迹" {
          tunnel: [_ w247] -> w95
          tunnel: w90 -> [_ w247]
          frame False {
          }
          frame True {
          }
        }
        n144 = case shown="真" "打开轨迹" {
          tunnel: [_ w248] -> w192
          tunnel: w92 -> [_ w248]
          frame False {
          }
          frame True {
          }
        }
        n145 = Array Size(array=w155) -> (size(s)=w157:i32)
        n146 = call "IMAQ Overlay Multiple Lines 2"("Image"=w93, "Line End Points"=w92, "Drawing Mode (Frame)"=w104, "Color"=u32 3071, "Width"=u32 5) -> ("Image Out"=→"中心轨迹和尖端轨迹":T2)  [unwired: 9 in, 1 out]
        n147 = Array Size(array=w151) -> (size(s)=w153:i32)
        n148 = Subtract(x=w157, y=1) -> (x-y=w156:i32)
        n149 = Subtract(x=w153, y=1) -> (x-y=w152:i32)
        n150 = Index Array "索引数组"(array=w155, index=w156) -> (element=w142:dbl)
        "now_end_point_x" <- w142
        n151 = Subtract "delta_x"(x=w142, y=w141) -> (x-y=w113:dbl)
        "delta_x" <- w113
        n152 = Build Array (concatenate) "delta_x"(w134, w113) -> (w132:dbl[])
        n153 = Square(x=w113) -> (x^2=w138:dbl)
        n154 = Index Array "索引数组"(array=w151, index=w152) -> (element=w139:dbl)
        "now_end_point_y" <- w139
        n155 = Subtract "delta_y"(x=w139, y=w140) -> (x-y=w112:dbl)
        "delta_y" <- w112
        n156 = Build Array (concatenate) "delta_y"(w133, w112) -> (w131:dbl[])
        n157 = Square(x=w112) -> (x^2=w137:dbl)
        n158 = Add(x=w138, y=w137) -> (x+y=w136:dbl)
        n159 = Square Root(x=w136) -> (sqrt(x)=w135:dbl)
        "delta_distance" <- w135
        n160 = Divide(x=w113, y=w112) -> (x/y=w111:dbl)
        "tan(v)" <- w111
        n161 = Divide(x=w135, y=w117) -> (x/y=w116:dbl)
        "delta_velocity" <- w116
        n162 = Build Array (concatenate)(w110, w111) -> (w109:dbl[])
        n163 = Build Array (concatenate) "delta_velocity"(w115, w116) -> (w114:dbl[])
        n164 = Build Array(w167, w166, w165, w164, w159, w163, w162, w161, w155, w151, w132, w131, w118, w114, w109, w101) -> (→"all parameters":dbl[][])
        "Numeric 5" <- w89
        "T" <- w89
        "T" <- w89
        "prev_end_point_x" <- w147
        "prev_end_point_y" <- w143
        "prev time" <- w126
      }
    }
    frame #3 {
      # "4. The error -314220 indicates that the other endpoint has been destroyed. The VI ignores this error."
      # "3. Destroy the stream endpoint when you click Stop or when an error occurs."
      # "Close"
      n165 = Flush Stream(8:w384, 11:w387) -> (0:w385:errorcluster, 3:w386:refnum<k21>)  [unwired: 2 in, 1 out]
      n166 = Destroy Stream Endpoint(8:w385, 11:w386) -> (0:w379:errorcluster)
      n167 = Unbundle By Name(w379) -> ("code"=w383:i32)
      n168 = xnode "Error Ring"() -> ("错误输出"=w380:errorcluster)
      n169 = Not Equal?(x=w383, y=-314220) -> (x != y?=w381:bool)
      n170 = Select(t=w379, s=w381, f=w380) -> (s? t:f=→"error out":errorcluster)
    }
  }
